vi "getTaskReqstQueue.vi"(8 "error in (no error)":errorcluster, 11 "TaskRef":refnum<vi>) -> (0 "error IO":errorcluster, 2 "TaskReqst_queue":refnum<queue>, 3 "TaskRef out":refnum<vi>)   [LabVIEW 2015, in "pdbm_task_route.lvlib"]
uses:
  pdbm_task_route.lvlib
  UsrDefine/TaskReqst.ctl
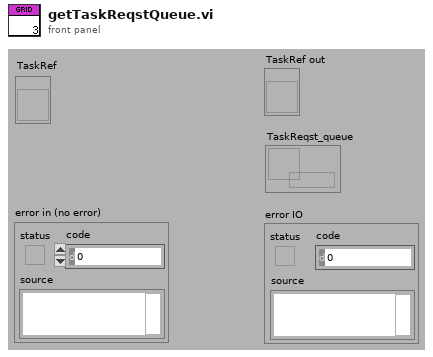
[diagram p1: front panel]
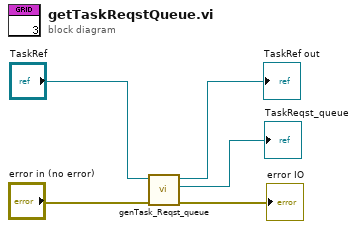
[diagram p0: block diagram]
diagram:
  n1 = call "genTask_Reqst_queue.vi"("error in (no error)"="error in (no error)", "TaskRef"="TaskRef") -> ("error IO"=→"error IO":errorcluster, "TaskReqst_queue"=→"TaskReqst_queue":refnum<queue>, "TaskRef out"=→"TaskRef out":refnum<vi>)  [unwired: 7 in]
